vi "电流方向控制-PLC.vi"() -> ()   [LabVIEW 2021]
panel:
  in  "?":bool
  in  "PLC地址":string="192.168.100.10"
  in  "电流方向控制":cluster{"正向":bool, "反向":bool}
  out "?":bool
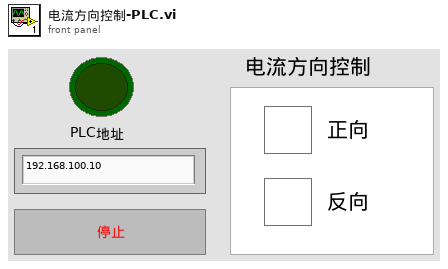
[diagram p1: front panel]
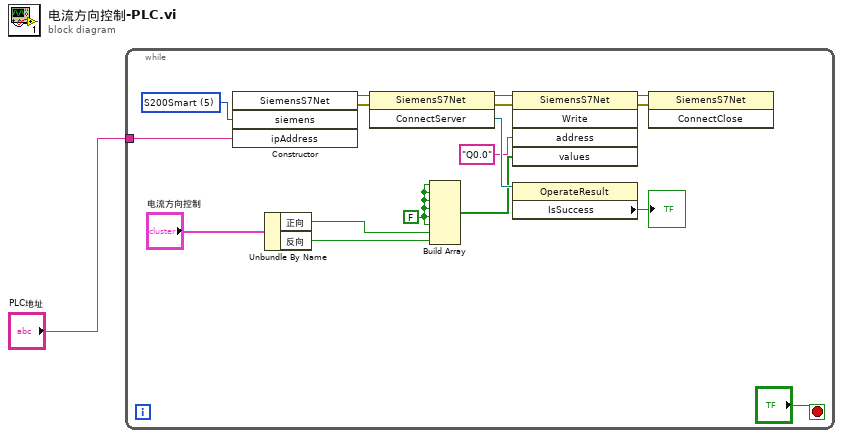
[diagram p0: block diagram]
diagram:
  n1 = while {
    tunnel: "PLC地址" -> [w2]
    stop <- "?" stop-if-true
    w4 = FALSE ("元素")
    w8 = 5 items=["S1200"=1, "S300"=2, "S400"=3, "S1500"=4, "S200Smart"=5, "S200"=6] ("siemens")
    n2 = constructor class="SiemensS7Net"("siemens"=w8, "ipAddress"=w2) -> (reference out=w17:refnum<k24>, error out=w18:errorcluster)  [unwired: 3 in, 3 out]
    n3 = Unbundle By Name("电流方向控制") -> ("正向"=w6:bool, "反向"=w5:bool)
    n4 = invoke class="SiemensS7Net" method="ConnectServer"(reference=w17, error in=w18) -> (reference out=w13:refnum<k24>, error out=w12:errorcluster, "ConnectServer"=w15:refnum<k24>)  [unwired: 1 in]
    n5 = Build Array(w4, w4, w4, w4, w4, w4, w6, w5) -> (w9:bool[])
    n6 = invoke class="SiemensS7Net" method="Write"(reference=w13, error in=w12, "address"="Q0.0", "values"=w9) -> (reference out=w10:refnum<k24>, error out=w11:errorcluster)  [unwired: 1 in, 3 out]
    n7 = property class="OperateResult"(reference=w15) -> ("IsSuccess"=→"?":bool)  [unwired: 1 in, 2 out]
    n8 = invoke class="SiemensS7Net" method="ConnectClose"(reference=w10, error in=w11) -> ()  [unwired: 1 in, 3 out]
  }
